vi "KernelConvolution.vi"(8 "error in":errorcluster, 9 "Pixel Co-ordinates":cluster{"x":i32, "y":i32}, 10 "Original Image":T2(plugin-control), 11 "matrix":T1=[[1.0, 1.0, 1.0], [1.0, 1.0, 1.0], [1.0, 1.0, 1.0]]) -> (0 "error out":errorcluster, 3 "NewPixelValues":T1=[[1.0, 1.0, 1.0], [1.0, 1.0, 1.0], [1.0, 1.0, 1.0]])   [LabVIEW 2017]
uses:
  <vilib>/Analysis/Matrix/Datatypes/RealMatrix.ctl
  <vilib>/Analysis/Matrix/Numeric/Multiply/Multiply - RM,RM.vi
  <vilib>/Analysis/Matrix/NI_Matrix.lvlib
  <vilib>/vision/NI_Vision_Development_Module.lvlib
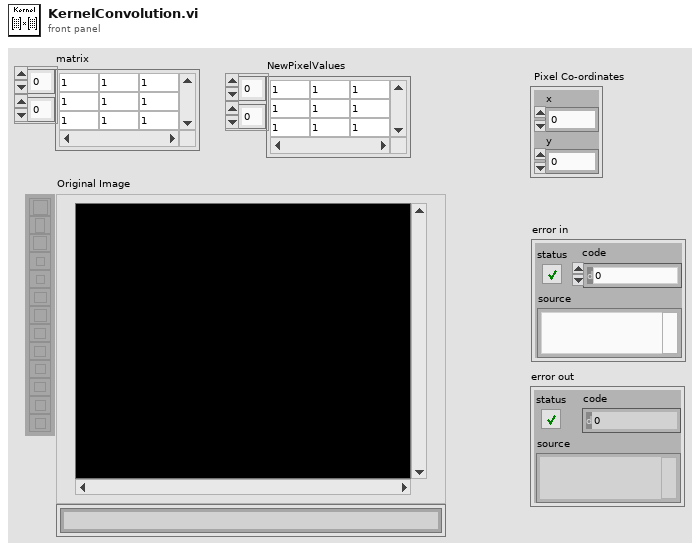
[diagram p1: front panel]
types:
  T1 = typedef "NI_Matrix.lvlib/RealMatrix.ctl" = dbl[][]
  T2 = typedef "IMAQ Image.ctl" = refnum<image>
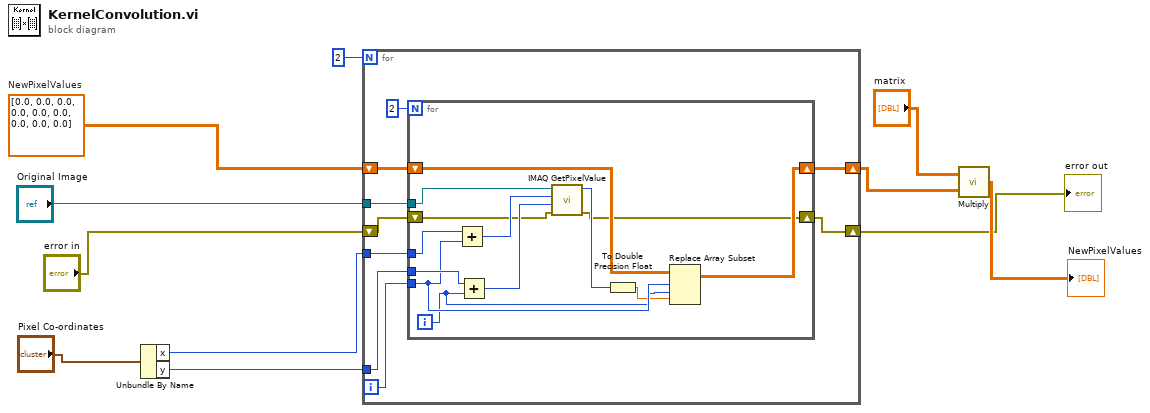
[diagram p0: block diagram]
diagram:
  w9 = T1 [[0.0, 0.0, 0.0], [0.0, 0.0, 0.0], [0.0, 0.0, 0.0]]  # NewPixelValues
  n1 = Unbundle By Name("Pixel Co-ordinates") -> ("x"=w2:i32, "y"=w1:i32)
  n2 = for {
    N: 2 -> [_]
    tunnel: w2 -> [w18]
    tunnel: "Original Image" -> [w17]
    shift-right: [w15] -> w7
    shift-left: w9 -> [w16]
    shift-right: [w13] -> w4
    shift-left: "error in" -> [w14]
    tunnel: w1 -> [w12]
    i -> [w19]
    n3 = for {
      N: 2 -> [_]
      tunnel: w19 -> [w28]
      tunnel: w18 -> [w33]
      tunnel: w12 -> [w32]
      tunnel: w17 -> [w29]
      shift-right: [w23] -> w15
      shift-left: w16 -> [w26]
      shift-right: [w21] -> w13
      shift-left: w14 -> [w22]
      i -> [w27]
      n4 = Add(x=w33, y=w28) -> (x+y=w31:i32)
      n5 = Add(x=w32, y=w27) -> (x+y=w30:i32)
      n6 = call "IMAQ GetPixelValue"("Image"=w29, "X Coordinate"=w31, "Y Coordinate"=w30, "error in (no error)"=w22) -> ("Pixel Value (U8)"=w25:u8, "error out"=w21:errorcluster)  [unwired: 2 in, 3 out]
      n7 = To Double Precision Float(number=w25) -> (double precision float=w24:dbl)
      n8 = Replace Array Subset(array=w26, new element=w24, index (row)=w28, index (col)=w27) -> (w23:T1)
    }
  }
  "error out" <- w4
  n9 = call-poly <vilib>:"Multiply.vi"("Real Matrix B"=w7, "Real Matrix A"="matrix") -> ("A * B"=→"NewPixelValues":T1)
